vi "file list -- accumulate.vi"(11 "file path":path=path "/snowfall/Users/arcadi/Desktop/Ultrasound/Experiment/YBCO_4/Round1/Sweep12/June_2011/062511/221.16400K_300_3100_001_062511.dat") -> (0 "timestamp":dbl[](array[numeric]), 2 "sweep file name array":T1[](array[typedef]), 3 "temperatures":dbl[](array[numeric]))   [LabVIEW 2010]
uses:
  sweep file name.ctl
  <vilib>/Utility/file.llb/Read From Spreadsheet File (string).vi
panel:
  in  "dummy 2":T1={"temperature"=0.0, "temperature str"="", "file path"=path "/snowfall/Users/arcadi/Desktop/Ultrasound/Experiment/YBCO_4/Round1/Sweep12/June_2011/062511/221.16400K_300_3100_001_062511.dat", "last mod"=timestamp(0 s since 1904-01-01), "file name str"="", "mod time(min)"=0.0, "file format"=enum.""}
  in  "sweep file name":T1={"temperature"=0.0, "temperature str"="", "file path"=path "/snowfall/Users/arcadi/Desktop/Ultrasound/Experiment/YBCO_4/Round1/Sweep12/June_2011/062511/221.16400K_300_3100_001_062511.dat", "last mod"=timestamp(0 s since 1904-01-01), "file name str"="", "mod time(min)"=0.0, "file format"=enum.""}
  in  "dummy":T1={"temperature"=0.0, "temperature str"="", "file path"=path "/snowfall/Users/arcadi/Desktop/Ultrasound/Experiment/YBCO_4/Round1/Sweep12/June_2011/062511/221.16400K_300_3100_001_062511.dat", "last mod"=timestamp(0 s since 1904-01-01), "file name str"="", "mod time(min)"=0.0, "file format"=enum.""}
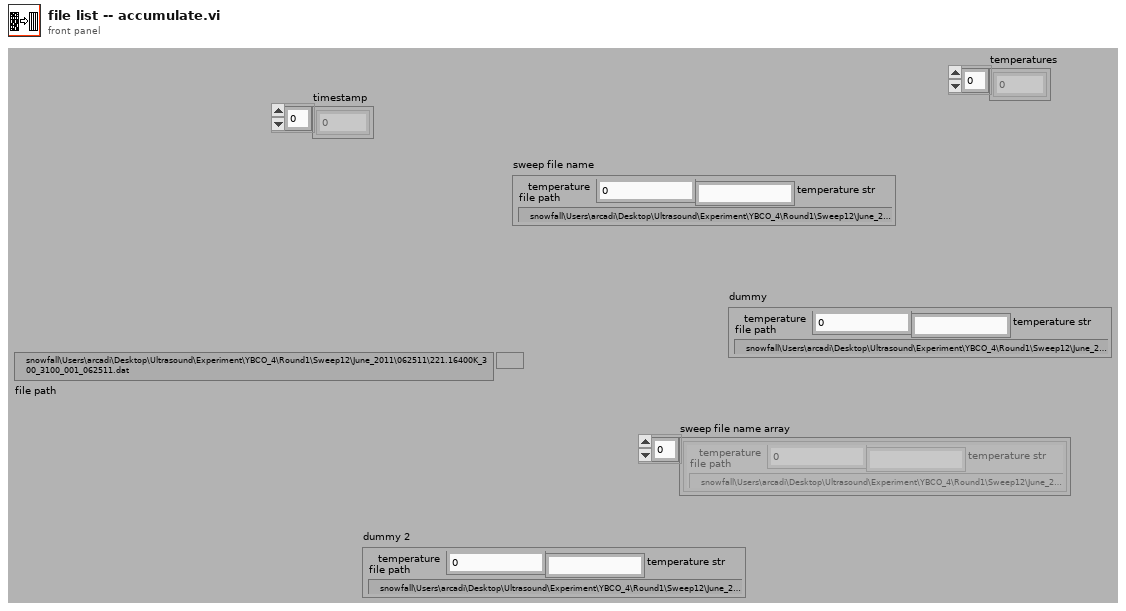
[diagram p1: front panel]
types:
  T1 = typedef "sweep file name.ctl" = cluster{"temperature":dbl, "temperature str":string, "file path":path, "last mod":timestamp, "file name str":string, "mod time(min)":dbl, "file format":enum16{"", "ascii", "binary"}}
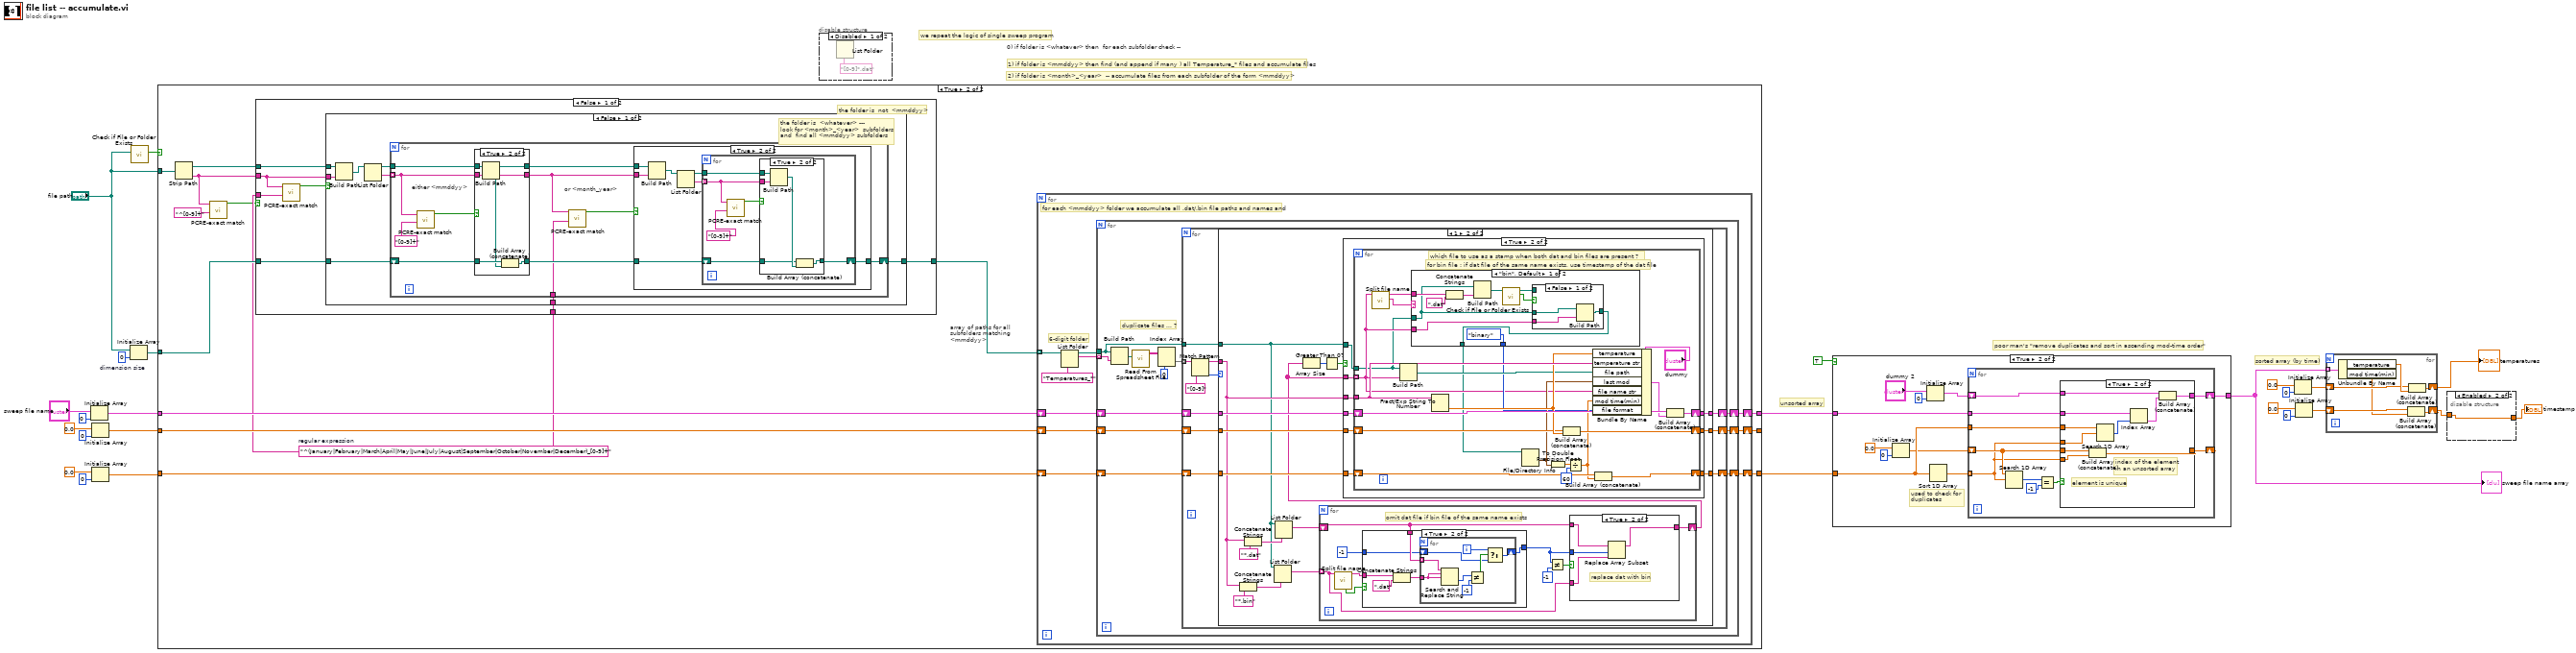
[diagram p0: block diagram]
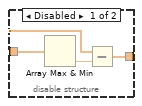
[diagram p2: hidden frame]
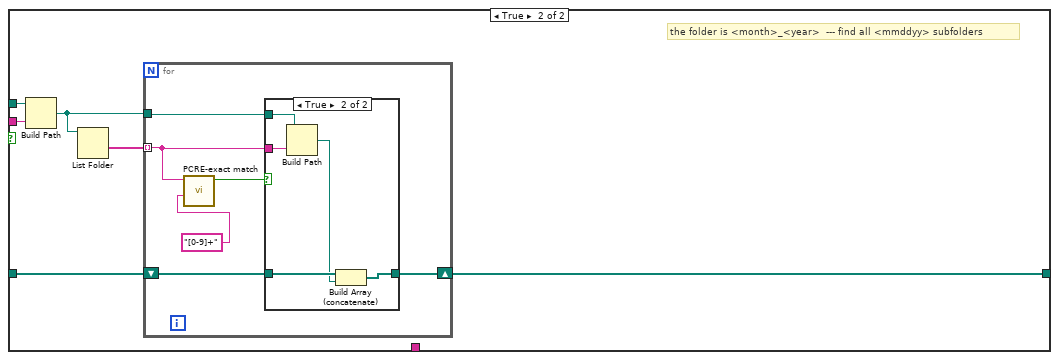
[diagram p10: hidden frame]
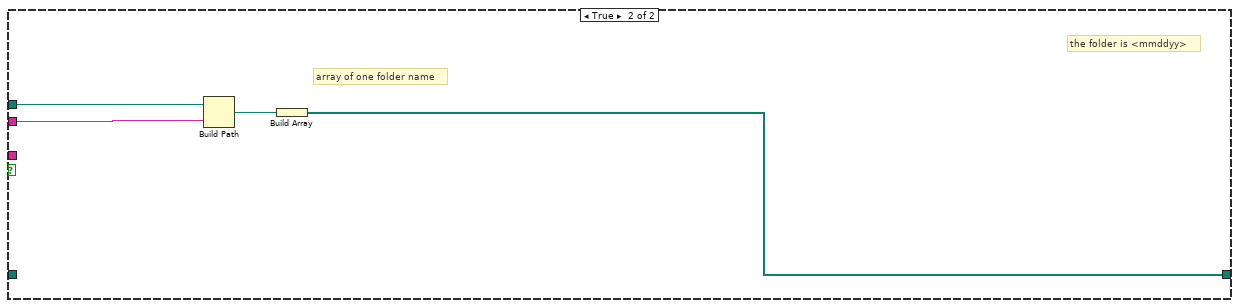
[diagram p12: hidden frame]
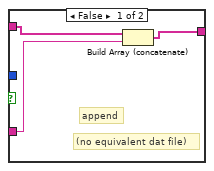
[diagram p14: hidden frame]
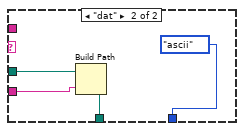
[diagram p18: hidden frame]
diagram:
  w3 = 0  # dimension size
  # "0) if folder is <whatever> then  for each subfolder check --"
  # "sorted array (by time)"
  # "unsorted array"
  # "poor man's \"remove duplicates and sort in ascending mod-time order\""
  # "1) if folder is <mmddyy> then find (and append if many ) all Temperature_* files and accumulate files"
  # "2) if folder is <month>_<year>  -- accumulate files from each subfolder of the form <mmddyy>"
  # "we repeat the logic of single sweep program"
  n1 = Initialize Array("sweep file name", 0 ("dimension size")) -> (w21:T1[])
  n2 = Initialize Array(0.0 ("dimension size"), 0 ("dimension size")) -> (w20:dbl[])
  n3 = Initialize Array(0.0 ("dimension size"), 0 ("dimension size")) -> (w17:dbl[])
  n4 = Initialize Array("file path", w3) -> (w1:path[])
  n5 = call <vilib>:"Check if File or Folder Exists.vi"("path"="file path") -> ("file or folder exists?"=w26:bool)  [unwired: 8 in, 2 out]
  n6 = case shown="True" w26 {
    tunnel: "file path" -> [_ w39]
    tunnel: [w29 w41] -> w14
    tunnel: [w28 w40] -> _
    tunnel: w21 -> [w29 w43]
    tunnel: w20 -> [w28 w42]
    tunnel: w17 -> [w27 w38]
    tunnel: [w27 w37] -> w15
    tunnel: w1 -> [_ w34]
    frame False {
    }
    frame True {
      w33 = "^(January|February|March|April|May|June|July|August|September|October|November|December)_[0-9]+"  # regular expression
      # "array of paths for all  \nsubfolders matching\n<mmddyy>"
      n7 = Strip Path(path=w39) -> (stripped path=w36:path, name=w32:string)
      n8 = call "PCRE-exact match.vi"("regular expression"="^[0-9]+", "input string"=w32) -> ("exact match"=w30:bool)  [unwired: 8 in, 1 out]
      n9 = case shown="False" w30 {
        tunnel: [w50 w118] -> w35
        tunnel: w36 -> [w49 w117]
        tunnel: w32 -> [w45 w116]
        tunnel: w33 -> [w46 _]
        tunnel: w34 -> [w48 _]
        tunnel: w33 -> [w47 _]
        frame False {
          # "the folder is  not  <mmddyy>"
          n10 = call "PCRE-exact match.vi"("regular expression"=w46, "input string"=w45) -> ("exact match"=w44:bool)  [unwired: 8 in, 1 out]
          n11 = case shown="False" w44 {
            tunnel: [w52 w101] -> w50
            tunnel: w45 -> [w55 w100]
            tunnel: w49 -> [w56 w99]
            tunnel: w48 -> [w54 w98]
            tunnel: w47 -> [w53 _]
            frame False {
              # "the folder is  <whatever> --- \nlook for <month>_<year>  subfolders \nand  find all <mmddyy> subfolders"
              n12 = Build Path(base path=w56, name or relative path=w55) -> (appended path=w57:path)
              n13 = List Folder(path=w57) -> (path out=w51:path, folder names=w58:string[])  [unwired: 3 in, 2 out]
              n14 = for {
                tunnel: w58 -> [w64] mode=indexing
                shift-right: [w68] -> w52
                shift-left: w54 -> [w69]
                tunnel: w51 -> [w66]
                tunnel: w53 -> [w60]
                # "or <month_year>"
                # "either <mmddyy>"
                n15 = call "PCRE-exact match.vi"("regular expression"="[0-9]+", "input string"=w64) -> ("exact match"=w62:bool)  [unwired: 8 in, 1 out]
                n16 = case shown="True" w62 {
                  tunnel: w66 -> [w90 w93]
                  tunnel: w64 -> [w91 w94]
                  tunnel: w69 -> [w92 w97]
                  tunnel: [w92 w95] -> w67
                  tunnel: [w91 w94] -> w61
                  tunnel: [w90 w93] -> w65
                  frame False {
                  }
                  frame True {
                    n17 = Build Path(base path=w93, name or relative path=w94) -> (appended path=w96:path)
                    n18 = Build Array (concatenate)(w97, w96) -> (w95:path[])
                  }
                }
                n19 = call "PCRE-exact match.vi"("regular expression"=w60, "input string"=w61) -> ("exact match"=w59:bool)  [unwired: 8 in, 1 out]
                n20 = case shown="True" w59 {
                  tunnel: [w70 w73] -> w68
                  tunnel: w67 -> [w70 w74]
                  tunnel: w65 -> [_ w77]
                  tunnel: w61 -> [_ w76]
                  frame False {
                  }
                  frame True {
                    n21 = Build Path(base path=w77, name or relative path=w76) -> (appended path=w72:path)
                    n22 = List Folder(path=w72) -> (path out=w71:path, folder names=w75:string[])  [unwired: 3 in, 2 out]
                    n23 = for {
                      tunnel: w75 -> [w80] mode=indexing
                      shift-right: [w82] -> w73
                      shift-left: w74 -> [w83]
                      tunnel: w71 -> [w81]
                      n24 = call "PCRE-exact match.vi"("regular expression"="[0-9]+", "input string"=w80) -> ("exact match"=w78:bool)  [unwired: 8 in, 1 out]
                      n25 = case shown="True" w78 {
                        tunnel: w83 -> [w84 w88]
                        tunnel: [w84 w87] -> w82
                        tunnel: w81 -> [_ w86]
                        tunnel: w80 -> [_ w85]
                        frame False {
                        }
                        frame True {
                          n26 = Build Path(base path=w86, name or relative path=w85) -> (appended path=w89:path)
                          n27 = Build Array (concatenate)(w88, w89) -> (w87:path[])
                        }
                      }
                    }
                  }
                }
              }
            }
            frame True {
              # "the folder is <month>_<year>  --- find all <mmddyy> subfolders"
              n28 = Build Path(base path=w99, name or relative path=w100) -> (appended path=w102:path)
              n29 = List Folder(path=w102) -> (folder names=w103:string[])  [unwired: 3 in, 3 out]
              n30 = for {
                tunnel: w103 -> [w106] mode=indexing
                shift-right: [w107] -> w101
                shift-left: w98 -> [w108]
                tunnel: w102 -> [w109]
                n31 = call "PCRE-exact match.vi"("regular expression"="[0-9]+", "input string"=w106) -> ("exact match"=w104:bool)  [unwired: 8 in, 1 out]
                n32 = case shown="True" w104 {
                  tunnel: w109 -> [_ w115]
                  tunnel: w106 -> [_ w114]
                  tunnel: w108 -> [w110 w113]
                  tunnel: [w110 w111] -> w107
                  frame False {
                  }
                  frame True {
                    n33 = Build Path(base path=w115, name or relative path=w114) -> (appended path=w112:path)
                    n34 = Build Array (concatenate)(w113, w112) -> (w111:path[])
                  }
                }
              }
            }
          }
        }
        frame True {
          # "the folder is <mmddyy>"
          # "array of one folder name"
          n35 = Build Path(base path=w117, name or relative path=w116) -> (appended path=w119:path)
          n36 = Build Array(w119) -> (w118:path[])
        }
      }
      n37 = for {
        tunnel: w35 -> [w125] mode=indexing
        shift-right: [w123] -> w41
        shift-left: w43 -> [w126]
        shift-right: [w124] -> w40
        shift-left: w42 -> [w122]
        shift-right: [w120] -> w37
        shift-left: w38 -> [w121]
        # "6-digit folder"
        # "for each <mmddyy> folder we accumulate all .dat/.bin file paths and names and"
        n38 = List Folder(path=w125, pattern="Temperatures_*") -> (filenames=w127:string[])  [unwired: 2 in, 3 out]
        n39 = for {
          tunnel: w127 -> [w131] mode=indexing
          tunnel: w125 -> [w139]
          shift-right: [w133] -> w123
          shift-left: w126 -> [w140]
          shift-right: [w138] -> w124
          shift-left: w122 -> [w132]
          shift-right: [w129] -> w120
          shift-left: w121 -> [w130]
          # "duplicate files ... ?"
          n40 = Build Path(base path=w139, name or relative path=w131) -> (appended path=w137:path)
          n41 = call-poly <vilib>:"Read From Spreadsheet File.vi"("file path (dialog if empty)"=w137) -> ("all rows"=w136:string[][])  [unwired: 6 in, 4 out]
          n42 = Index Array(array=w136, index (col)=0 ("disabled index (col)")) -> (element=w134:string[])  [unwired: 1 in]
          n43 = for {
            tunnel: w134 -> [w145] mode=indexing
            tunnel: w139 -> [w150]
            shift-right: [w148] -> w133
            shift-left: w140 -> [w149]
            shift-right: [w146] -> w138
            shift-left: w132 -> [w147]
            shift-right: [w141] -> w129
            shift-left: w130 -> [w142]
            n44 = Match Pattern(string=w145, regular expression="[0-9]") -> (offset past match=w143:i32)  [unwired: 1 in, 3 out]
            n45 = case shown="1" w143 {
              tunnel: w150 -> [_ w157]
              tunnel: w145 -> [_ w158]
              tunnel: w149 -> [w152 w168]
              tunnel: [w152 w167] -> w148
              tunnel: w147 -> [w153 w166]
              tunnel: [w153 w165] -> w146
              tunnel: w142 -> [w151 w164]
              tunnel: [w151 w163] -> w141
              frame -1, Default {
              }
              frame 1 {
                n46 = Concatenate Strings(w158, "*.bin" ("string")) -> (w159:string)
                n47 = Concatenate Strings(w158, "*.dat" ("string")) -> (w169:string)
                n48 = List Folder(path=w157, pattern=w159) -> (filenames=w154:string[])  [unwired: 2 in, 3 out]
                n49 = List Folder(path=w157, pattern=w169) -> (filenames=w156:string[])  [unwired: 2 in, 3 out]
                n50 = for {
                  shift-right: [w173] -> w155
                  shift-left: w156 -> [w174]
                  tunnel: w154 -> [w172] mode=indexing
                  # "omit dat file if bin file of the same name exists"
                  n51 = call "Split file name.vi"("file name"=w172) -> ("name"=w178:string, "exact match"=w179:bool)  [unwired: 8 in, 1 out]
                  n52 = case shown="True" w179 {
                    tunnel: w178 -> [_ w192]
                    tunnel: w174 -> [_ w191]
                    tunnel: [w187 w189] -> w171
                    tunnel: -1 -> [w187 w188]
                    frame False {
                    }
                    frame True {
                      n53 = Concatenate Strings(w192, ".dat" ("string")) -> (w190:string)
                      n54 = for {
                        tunnel: w191 -> [w201] mode=indexing
                        tunnel: w190 -> [w200]
                        shift-right: [w194] -> w189
                        shift-left: w188 -> [w195]
                        i -> [w196]
                        n55 = Search and Replace String(input string=w201, search string=w200, replace string=w200) -> (offset past replacement=w198:i32)  [unwired: 5 in, 3 out]
                        n56 = Not Equal?(x=w198, y=-1) -> (x != y?=w199:bool)
                        n57 = Select(t=w196, s=w199, f=w195) -> (s? t:f=w194:i32)
                      }
                    }
                  }
                  n58 = Not Equal?(x=w171, y=-1) -> (x != y?=w175:bool)
                  n59 = case shown="True" w175 {
                    tunnel: w174 -> [w182 w186]
                    tunnel: [w181 w183] -> w173
                    tunnel: w172 -> [w180 w185]
                    tunnel: w171 -> [_ w184]
                    frame False {
                      # "(no equivalent dat file)"
                      # "append"
                      n60 = Build Array (concatenate)(w182, w180) -> (w181:string[])
                    }
                    frame True {
                      # "replace dat with bin"
                      n61 = Replace Array Subset(array=w186, new element=w185, index=w184) -> (w183:string[])
                    }
                  }
                }
                n62 = Array Size(array=w155) -> (size(s)=w162:i32)
                n63 = Greater Than 0?(x=w162) -> (x > 0?=w161:bool)
                n64 = case shown="True" w161 {
                  tunnel: w155 -> [_ w213]
                  tunnel: w157 -> [_ w212]
                  tunnel: w158 -> [_ w211]
                  tunnel: w168 -> [w204 w210]
                  tunnel: [w204 w207] -> w167
                  tunnel: w166 -> [w203 w209]
                  tunnel: [w203 w206] -> w165
                  tunnel: w164 -> [w202 w208]
                  tunnel: [w202 w205] -> w163
                  frame False {
                    # "duplicat tempearture folder"
                  }
                  frame True {
                    n65 = for {
                      tunnel: w213 -> [w217] mode=indexing
                      tunnel: w212 -> [w216]
                      tunnel: w211 -> [w233]
                      shift-right: [w225] -> w207
                      shift-left: w210 -> [w232]
                      shift-right: [w224] -> w206
                      shift-left: w209 -> [w229]
                      shift-right: [w223] -> w205
                      shift-left: w208 -> [w227]
                      # "which file to use as a stamp when both dat and bin files are present ?"
                      # "for bin file : if dat file of the same name exists, use timestamp of the dat file"
                      n66 = call "Split file name.vi"("file name"=w217) -> ("extension"=w218:string, "name"=w214:string)  [unwired: 8 in, 1 out]
                      n67 = Build Path(base path=w216, name or relative path=w217) -> (appended path=w228:path)
                      n68 = case shown="\"bin\", Default" w218 {
                        tunnel: [enum16{"", "ascii", "binary"}."binary" ("action") enum16{"", "ascii", "binary"}."ascii" ("action")] -> w219
                        tunnel: w217 -> [w235 w251]
                        tunnel: w216 -> [w236 w250]
                        tunnel: [w238 w249] -> w215
                        tunnel: w214 -> [w242 _]
                        frame "bin", Default {
                          n69 = Concatenate Strings(w242, ".dat" ("string")) -> (w240:string)
                          n70 = Build Path(base path=w236, name or relative path=w240) -> (appended path=w239:path)
                          n71 = call <vilib>:"Check if File or Folder Exists.vi"("path"=w239) -> ("file or folder exists?"=w241:bool, "dup path"=w237:path)  [unwired: 8 in, 1 out]
                          n72 = case shown="False" w241 {
                            tunnel: [w245 w248] -> w238
                            tunnel: w237 -> [_ w248]
                            tunnel: w236 -> [w247 _]
                            tunnel: w235 -> [w246 _]
                            frame False {
                              n73 = Build Path(base path=w247, name or relative path=w246) -> (appended path=w245:path)
                            }
                            frame True {
                            }
                          }
                        }
                        frame "dat" {
                          n74 = Build Path(base path=w250, name or relative path=w251) -> (appended path=w249:path)
                        }
                      }
                      n75 = Fract/Exp String To Number(string=w233) -> (number=w230:dbl)  [unwired: 3 in, 1 out]
                      n76 = File/Directory Info(path=w215) -> (last mod=w226:timestamp)  [unwired: 1 in, 6 out]
                      n77 = To Double Precision Float(number=w226) -> (double precision float=w222:dbl)
                      n78 = Build Array (concatenate)(w229, w230) -> (w224:dbl[])
                      n79 = Divide(x=w222, y=60) -> (x/y=w220:dbl)
                      n80 = Bundle By Name(cluster="dummy", "temperature"=w230, "temperature str"=w233, "file path"=w228, "last mod"=w226, "file name str"=w217, "mod time(min)"=w220, "file format"=w219) -> (w231:T1)
                      n81 = Build Array (concatenate)(w227, w220) -> (w223:dbl[])
                      n82 = Build Array (concatenate)(w232, w231) -> (w225:T1[])
                    }
                  }
                }
              }
            }
          }
        }
      }
    }
  }
  n83 = disable-structure shown="Disabled" {
    frame Disabled {
      n84 = List Folder(pattern="[0-9]*.dat") -> ()  [unwired: 3 in, 4 out]
    }
    frame Enabled {
    }
  }
  n85 = case shown="True" TRUE {
    tunnel: w15 -> [_ w258]
    tunnel: w14 -> [w254 w263]
    tunnel: [w254 w262] -> w4
    frame False {
    }
    frame True {
      # "used to check for \nduplicates"
      n86 = Initialize Array(0.0 ("dimension size"), 0 ("dimension size")) -> (w255:dbl[])
      n87 = Initialize Array("dummy 2", 0 ("dimension size")) -> (w259:T1[])
      n88 = Sort 1D Array(array=w258) -> (sorted array=w264:dbl[])
      n89 = for {
        shift-right: [w271] -> w262
        shift-left: w259 -> [w270]
        shift-right: [w269] -> _
        shift-left: w255 -> [w268]
        tunnel: w264 -> [w265] mode=indexing
        tunnel: w258 -> [w267]
        tunnel: w263 -> [w266]
        n90 = Search 1D Array(1D array=w268, element=w265) -> (index of element=w274:i32)  [unwired: 1 in]
        n91 = Equal?(x=w274, y=-1) -> (x = y?=w272:bool)
        n92 = case shown="True" w272 {
          tunnel: [w276 w285] -> w271
          tunnel: w270 -> [w276 w286]
          tunnel: [w275 w277] -> w269
          tunnel: w268 -> [w275 w279]
          tunnel: w267 -> [_ w284]
          tunnel: w265 -> [_ w283]
          tunnel: w266 -> [_ w281]
          tunnel: w265 -> [_ w278]
          frame False {
            # "element is not unique"
          }
          frame True {
            # "index of the element \nin an unsorted array"
            # "element is unique"
            n93 = Build Array (concatenate)(w279, w278) -> (w277:dbl[])
            n94 = Search 1D Array(1D array=w284, element=w283) -> (index of element=w282:i32)  [unwired: 1 in]
            n95 = Index Array(array=w281, index=w282) -> (element=w280:T1)
            n96 = Build Array (concatenate)(w286, w280) -> (w285:T1[])
          }
        }
      }
    }
  }
  "sweep file name array" <- w4
  n97 = Initialize Array(0.0 ("dimension size"), 0 ("dimension size")) -> (w11:dbl[])
  n98 = Initialize Array(0.0 ("dimension size"), 0 ("dimension size")) -> (w8:dbl[])
  n99 = for {
    tunnel: w4 -> [w293] mode=indexing
    shift-right: [w287] -> w7
    shift-left: w11 -> [w291]
    shift-right: [w288] -> w6
    shift-left: w8 -> [w290]
    n100 = Unbundle By Name(w293) -> ("temperature"=w292:dbl, "mod time(min)"=w289:dbl)
    n101 = Build Array (concatenate)(w290, w289) -> (w288:dbl[])
    n102 = Build Array (concatenate)(w291, w292) -> (w287:dbl[])
  }
  "temperatures" <- w7
  n103 = disable-structure shown="Enabled" {
    disable-tunnel: w6 -> [w295 w297]
    disable-tunnel: [w294 w297] -> w5
    frame Disabled {
      n104 = Array Max & Min(array=w295) -> (min value=w296:dbl)  [unwired: 3 out]
      n105 = Subtract(x=w295, y=w296) -> (x-y=w294:dbl[])
    }
    frame Enabled {
    }
  }
  "timestamp" <- w5
